vi "InvMP_Host_flatpotential.vi"() -> ()   [LabVIEW 2019]
uses:
  <vilib>/rvi/interface/nirviMethod/nirviMethod.xnode
  <vilib>/rvi/errors/niLvFpgaMergeErrorWithErrorCode.vi
  <vilib>/rvi/interface/nirviReadWriteControl/nirviReadWriteControl.xnode
  <vilib>/rvi/interface/Simulation/niFpgaSimulationCallBeginRW.vi
  <vilib>/rvi/errors/niLvFpgaAdjustHostInterfaceError.vi
  <vilib>/Utility/file.llb/Write Delimited Spreadsheet (DBL).vi
  <vilib>/Analysis/NI_AALBase.lvlib
  <vilib>/Analysis/baseanly.llb/Mean (DBL).vi
  <vilib>/FPGAPlugInAG/Dynamic/niLvFpga_Reset_Dynamic.vi
  <vilib>/FPGAPlugInAG/Dynamic/niLvFpga_Run_Dynamic.vi
  <vilib>/rvi/interface/nirviCloseFPGA/nirviCloseFPGA.xnode
  <vilib>/rvi/interface/nirviOpenFPGA/nirviOpenFPGA.xnode
  <vilib>/FPGAPlugInAG/Dynamic/niLvFpga_ConfigureFifo_Dynamic.vi
  <vilib>/FPGAPlugInAG/Dynamic/niLvFpga_StartFifo_Dynamic.vi
  <vilib>/FPGAPlugInAG/Dynamic/niLvFpga_ReadFifo_Dynamic.vi
  <vilib>/FPGAPlugInAG/Dynamic/niLvFpga_StopFifo_Dynamic.vi
  <vilib>/FPGAPlugInAG/Dynamic/niLvFpga_Close_Dynamic.vi
panel:
  in  "Menu Ring":u16(ring) items=["No FB", "HW", "FB"]
  out "Fx out":sgl=5.0307837
  in  "wait time":sgl=50.0
  in  "Fiting Control":enum32{"Fitting Control", "Fitting Errors"}(tab)
  out "signal\n offset_X":sgl=5.0
  in  "Fit?":bool
  out "best fit parameters":sgl[](array[numeric])=[0.33487067, 59.390804, 36.828644, -192.99852, -9974.326, 113441.81]
  out "residue":dbl
  in  "initial\nparameters":dbl[](array[numeric])=[0.0, 65.0, 0.0, -747.0, 30000.0, 300000.0, 0.0]
  in  "Offset":sgl=5.0
  out "Fitting in \nprogress":bool
  in  "Cal px/V":dbl=93.535 format="%#_13g"
  out "Pos array":sgl[](array[numeric])
  out "Volt":sgl[](array[numeric])
  out "error out":errorcluster
  out "smoothing error":i32
  in  "Calibration":T1={"K0"=0.0, "K1"=1.0, "K2"=0.0, "K3"=0.0, "K4"=0.0, "K5"=0.0}
  in  "Use Cal?":bool=TRUE
  in  "V_offset":sgl
  in  "Bias":sgl=0.0001
  in  "Xmin":sgl=-1.0
  in  "Fmax":sgl=100.0
  in  "Xmax":sgl=3.0
  out "num of protocols":sgl=1592.0
  in  "Calibration ON/OFF":bool=TRUE
  in  "Xoffset":sgl=0.00147
  in  "Yoffset":sgl=-0.00294
  in  "sum_offset":sgl=-0.0068
  in  "DW":cluster{"xm":sgl, "Eb":sgl, "Tau":sgl, "dE":sgl}={"xm"=0.5, "Eb"=0.005, "Tau"=80.0, "dE"=0.0} {"dE" format="%#_3g"}
  in  "DL_Y":dbl=2.5 format="%#_13g"
  in  "TL_Y":dbl=2.5 format="%#_13g"
  in  "STOP":bool
  in  "FB time":u32=10
  in  "Triangle wave":T2={"signal offset_X"=5.0, "Scale X"=0.0, "signal offset_Y"=5.0, "Scale Y"=0.0, "Phase Shift"=40}
  in  "Elements":u32=100000
  in  "Data length":dbl=20.0
  out "Done saving":bool
  out "?":dbl=-187.0
  in  "Save Data":bool
  in  "mobX(px/V)":sgl=1.0
  in  "1/Xcali":sgl=1.0
  in  "DX":sgl=51.12
  out "Feedback Loop time":sgl=10.0 format="%.2f"
  out "Underflow":bool
  out "X":waveform(dbl)(graph)={"t0"=timestamp(0 s since 1904-01-01), "dt"=9.999999747378752e-06, "Y"=array[100000 elements]}
  out "Y":waveform(dbl)(graph)={"t0"=timestamp(0 s since 1904-01-01), "dt"=9.999999747378752e-06, "Y"=array[100000 elements]}
  out "Sum":waveform(dbl)(graph)={"t0"=timestamp(0 s since 1904-01-01), "dt"=9.999999747378752e-06, "Y"=array[100000 elements]}
  in  "Reaverage PS":bool
  out "meanX":dbl=0.16896048917708206 format="%0.5f"
  in  "Xmean":sgl
  out "PSX":dynamicdata(graph)=[{"t0"=timestamp(0 s since 1904-01-01), "dt"=1.0000000252621255, "Y"=array[50000 elements], "attributes"=variant("NI_ChannelName"=variant(string "PSD"))}]
  out "PSY":dynamicdata(graph)=[{"t0"=timestamp(0 s since 1904-01-01), "dt"=1.0000000252621255, "Y"=array[50000 elements], "attributes"=variant("NI_ChannelName"=variant(string "PSD"))}]
  out "PSsum":dynamicdata(graph)=[{"t0"=timestamp(0 s since 1904-01-01), "dt"=1.0000000252621255, "Y"=array[50000 elements], "attributes"=variant("NI_ChannelName"=variant(string "PSD"))}]
  out "Saveloop":u32
  in  "Feedback parameters":T3={"SP_QPDX"=0.0, "alpha"=-0.1, "ktrap"=45.7534, "alphacounterX"=0.0218689}
  in  "TW freq":dbl=1.0
  in  "Normalize signal":bool=TRUE
  out "meanY":dbl=0.4494399424203283 format="%0.5f"
  out "meanZ":dbl=0.6937766502952576 format="%0.4f"
  out "?":errorcluster
  in  "file path (dialog if empty)":path=path "C:/Users/Diffusivity/Desktop/Inverse_Mpemba_starting June16/26-08-2020/t.txt"
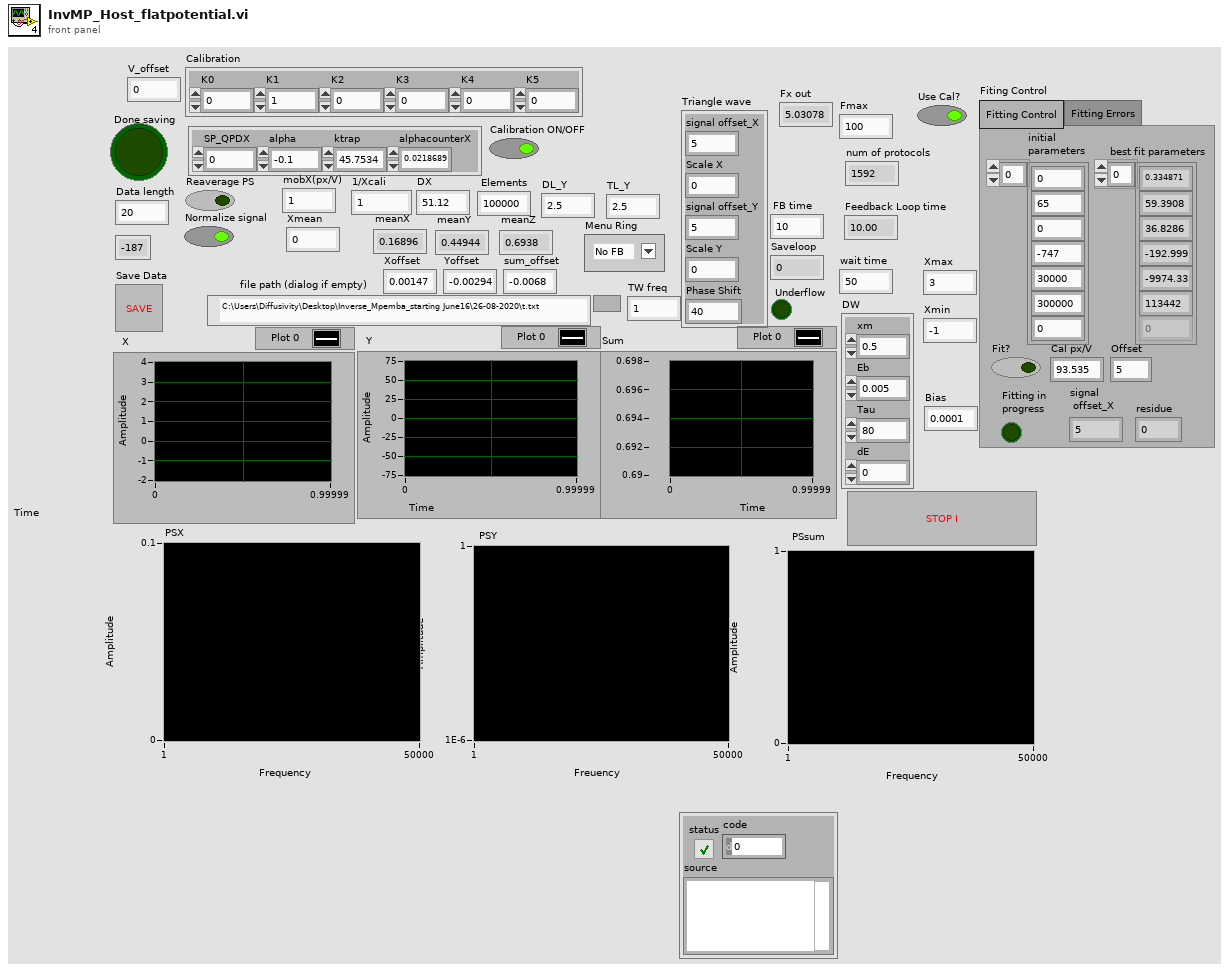
[diagram p1: front panel]
types:
  T1 = cluster{"K0":sgl, "K1":sgl, "K2":sgl, "K3":sgl, "K4":sgl, "K5":sgl}
  T2 = cluster{"signal offset_X":sgl, "Scale X":sgl, "signal offset_Y":sgl, "Scale Y":sgl, "Phase Shift":u32}
  T3 = cluster{"SP_QPDX":sgl, "alpha":sgl, "ktrap":sgl, "alphacounterX":sgl}
  T4 = cluster{"signal offset_X":sgl, "Scale X":sgl, "signal offset_Y":sgl, "Scale Y":sgl, u32}
  T5 = cluster{"[0]":sgl, "[1]":sgl, "[2]":sgl, "[3]":sgl, "[4]":sgl, "[5]":sgl}
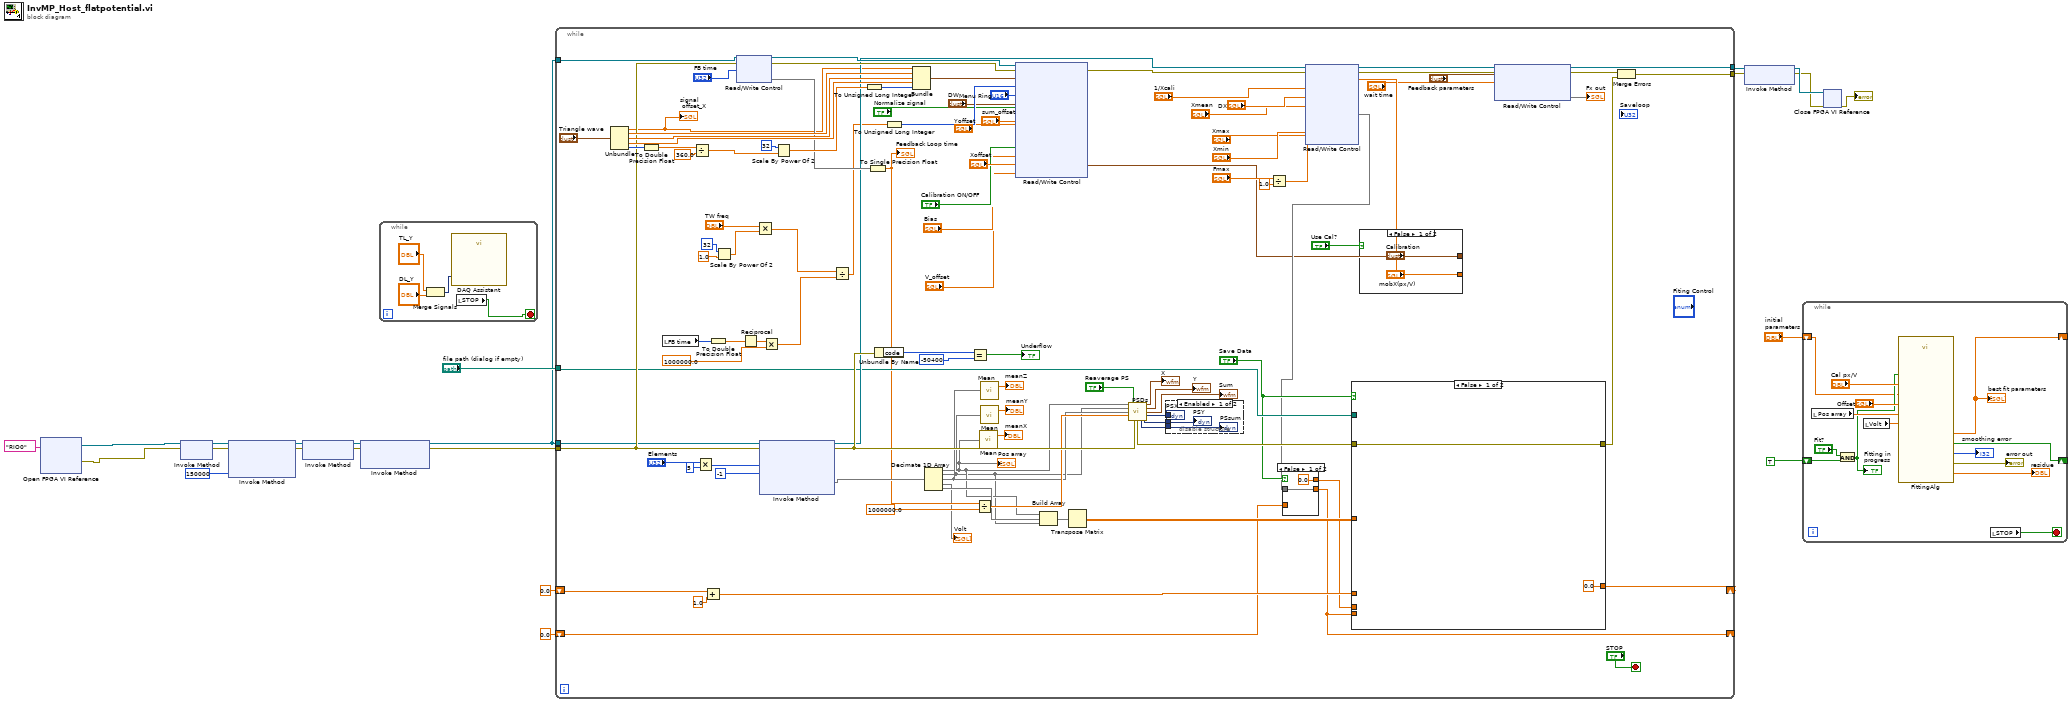
[diagram p0: block diagram]
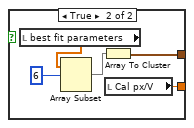
[diagram p2: hidden frame]
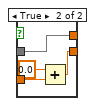
[diagram p3: hidden frame]
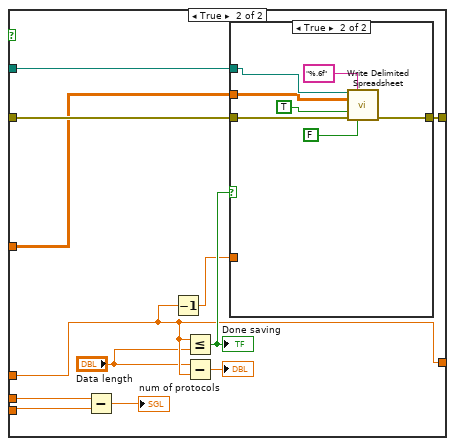
[diagram p5: hidden frame]
diagram:
  n1 = xnode "Open FPGA VI Reference"("resource name"=tag "RIO0") -> ("FPGA VI Reference Out"=w3:refnum<k20>, "error out"=w2:errorcluster)  [unwired: 1 in]
  n2 = xnode "Invoke Method"("FPGA VI Reference In"=w3, "error in"=w2) -> ("FPGA VI Reference Out"=w12:refnum<k20>, "error out"=w11:errorcluster)
  n3 = xnode "Invoke Method"("FPGA VI Reference In"=w12, "error in"=w11, "Requested Depth"=u32 150000) -> ("FPGA VI Reference Out"=w17:refnum<k20>, "error out"=w16:errorcluster)  [unwired: 1 out]
  n4 = xnode "Invoke Method"("FPGA VI Reference In"=w17, "error in"=w16) -> ("FPGA VI Reference Out"=w19:refnum<k20>, "error out"=w18:errorcluster)
  n5 = xnode "Invoke Method"("FPGA VI Reference In"=w19, "error in"=w18) -> ("FPGA VI Reference Out"=w15:refnum<k20>, "error out"=w14:errorcluster)  [unwired: 1 in]
  n6 = while {
    stop <- w23 stop-if-true
    n7 = Merge Signals("TL_Y", "DL_Y") -> (w26:dynamicdata)
    n8 = call "DAQ Assistant"("data"=w26) -> ()  [unwired: 17 in, 2 out]
    n9 = local read "STOP"() -> (w23:bool)
  }
  n10 = while {
    tunnel: w15 -> [w106]
    tunnel: w14 -> [w107]
    tunnel: "file path (dialog if empty)" -> [w76]
    tunnel: [w99] -> w21
    tunnel: [w112] -> w20
    tunnel: w15 -> [w94]
    shift-right: [w103] -> _
    shift-left: 0.0 -> [w102]
    shift-right: [w45] -> _
    shift-left: sgl 0.0 ("num of cycles") -> [w47]
    stop <- "STOP" stop-if-true
    n11 = Unbundle("Triangle wave") -> ("signal offset_X"=w33:sgl, "Scale X"=w116:sgl, "signal offset_Y"=w115:sgl, "Scale Y"=w114:sgl, "Phase Shift"=w117:u32)
    "signal\n offset_X" <- w33
    n12 = To Double Precision Float(number=w117) -> (double precision float=w123:dbl)
    n13 = local read "FB time"() -> (w66:u32)
    n14 = Divide(x=w123, y=360.0) -> (x/y=w121:dbl)
    n15 = Multiply(x="Elements", y=u32 5) -> (x*y=w108:u32)
    n16 = Add(x=w102, y=1.0) -> (x+y=w104:dbl)
    n17 = To Double Precision Float(number=w66) -> (double precision float=w67:dbl)
    n18 = Scale By Power Of 2(n=i16 32, x=1.0) -> (x*2^n=w71:dbl)
    n19 = xnode "Read/Write Control"("FPGA VI Reference In"=w106, "error in"=w107, "FB Time"="FB time") -> ("FPGA VI Reference Out"=w128:refnum<k20>, "error out"=w95:errorcluster, "FB Time"=w93)
    n20 = Reciprocal(x=w67) -> (1/x=w68:dbl)
    n21 = Multiply(x="TW freq", y=w71) -> (x*y=w64:dbl)
    n22 = xnode "Invoke Method"("FPGA VI Reference In"=w94, "error in"=w107, "Number of Elements"=w108, "Timeout (ms)"=-1) -> ("FPGA VI Reference Out"=w78:refnum<k20>, "error out"=w91:errorcluster, "Data"=w87:void[])  [unwired: 1 out]
    n23 = Multiply(x=w68, y=1000000.0) -> (x*y=w63:dbl)
    n24 = Scale By Power Of 2(n=i16 32, x=w121) -> (x*2^n=w119:dbl)
    n25 = Divide(x=w64, y=w63) -> (x/y=w62:dbl)
    n26 = To Unsigned Long Integer(number=w119) -> (unsigned 32bit integer=w113:u32)
    n27 = To Single Precision Float(number=w93) -> (single precision float=w73:sgl)
    "Feedback Loop time" <- w73
    n28 = Unbundle By Name(w91) -> ("code"=w111:i32)
    n29 = To Unsigned Long Integer(number=w62) -> (unsigned 32bit integer=w61:u32)
    n30 = Bundle("signal offset_X"=w33, "Scale X"=w116, "signal offset_Y"=w115, "Scale Y"=w114, w113) -> (w74:T4)  [unwired: 1 in]
    n31 = Decimate 1D Array(w87) -> (w35:void[], w27:void[], w54:void[], →"Volt":void[], w55:void[])
    "Pos array" <- w35
    n32 = Equal?(x=w111, y=-50400) -> (x = y?=→"Underflow":bool)
    n33 = Divide(x=w73, y=sgl 1000000.0) -> (x/y=w56:sgl)
    n34 = call-poly <vilib>:"Mean.vi"("X"=w35) -> ("mean"=→"meanX":dbl)  [unwired: 1 out]
    n35 = call-poly <vilib>:"Mean.vi"("X"=w54) -> ("mean"=→"meanZ":dbl)  [unwired: 1 out]
    n36 = call-poly <vilib>:"Mean.vi"("X"=w27) -> ("mean"=→"meanY":dbl)  [unwired: 1 out]
    n37 = Build Array(w35, w55, w27) -> (w97:void[])
    n38 = Transpose Matrix(1:w97) -> (0:w126:dbl[][])
    n39 = call "PSDs.vi"("X"=w35, "averaging done"="Reaverage PS", "Y"=w27, "sum"=w54, "dt"=w56, "error in (no error)"=w91) -> ("X"=→"X":waveform(dbl), "Y"=→"Y":waveform(dbl), "Sum"=→"Sum":waveform(dbl), "PSDX"=w83:dynamicdata, "error out"=w90:errorcluster, "PSDsum"=w81:dynamicdata, "PSDY"=w82:dynamicdata)  [unwired: 3 in]
    n40 = disable-structure shown="Enabled" {
      disable-tunnel: w83 -> [w146 _]
      disable-tunnel: w82 -> [w145 _]
      disable-tunnel: w81 -> [w144 _]
      frame Enabled {
        "PSX" <- w146
        "PSY" <- w145
        "PSsum" <- w144
      }
      frame Disabled {
      }
    }
    n41 = Divide(x="Fmax", y=sgl 1.0) -> (x/y=w42:sgl)
    n42 = case shown="False" "Use Cal?" {
      tunnel: ["Calibration" w137] -> w37
      tunnel: ["mobX(px/V)" w134] -> w36
      frame False {
      }
      frame True {
        n43 = local read "best fit parameters"() -> (w133:sgl[])
        n44 = Array Subset(array=w133, length=6) -> (w135:sgl[])  [unwired: 1 in]
        n45 = Array To Cluster(array=w135) -> (cluster=w137:T5)
        n46 = local read "Cal px/V"() -> (w134:dbl)
      }
    }
    n47 = xnode "Read/Write Control"("FPGA VI Reference In"=w128, "error in"=w95, "Triangle wave"=w74, "Frequency"=w61, "Enum"="Menu Ring", "DW"="DW", "Normalize signal"="Normalize signal", "sum_offset"="sum_offset", "Yoffset"="Yoffset", "Xoffset"="Xoffset", "Calibration ON/OFF"="Calibration ON/OFF", "Bias"="Bias", "Calibration"=w37, "V_offset"="V_offset") -> ("error out"=w77:errorcluster)  [unwired: 1 out]
    n48 = xnode "Read/Write Control"("FPGA VI Reference In"=w78, "error in"=w77, "MobX(px/V)"=w36, "1/Xcali"="1/Xcali", "DX"="DX", "Xmean"="Xmean", "Fmax"=w42, "Xmin"="Xmin", "Xmax"="Xmax") -> ("FPGA VI Reference Out"=w101:refnum<k20>, "error out"=w100:errorcluster, "num of cycles"=w44)
    n49 = case shown="False" "Save Data" {
      tunnel: w44 -> [w139 w140]
      tunnel: [w139 w141] -> w45
      tunnel: w47 -> [_ w142]
      tunnel: [sgl 0.0 ("num of cycles") w140] -> w46
      frame False {
      }
      frame True {
        n50 = Add(x=sgl 0.0 ("num of cycles"), y=w142) -> (x+y=w141:sgl)
      }
    }
    n51 = case shown="False" "Save Data" {
      tunnel: w126 -> [_ w155]
      tunnel: w76 -> [_ w160]
      tunnel: w90 -> [w148 w159]
      tunnel: [w148 w158] -> w125
      tunnel: w104 -> [_ w154]
      tunnel: [0.0 w154] -> w103
      tunnel: w46 -> [_ w151]
      tunnel: w45 -> [_ w150]
      frame False {
      }
      frame True {
        n52 = Subtract(x=w151, y=w150) -> (x-y=→"num of protocols":sgl)
        n53 = Decrement(x=w154) -> (x-1=w153:dbl)
        n54 = Less Or Equal?(x=w154, y="Data length") -> (x <= y?=w157:bool)
        "Done saving" <- w157
        n55 = Subtract(x="Data length", y=w154) -> (x-y=→"?":dbl)
        n56 = case shown="True" w157 {
          tunnel: w155 -> [_ w162]
          tunnel: w160 -> [_ w163]
          tunnel: w159 -> [w161 w166]
          tunnel: [w161 w165] -> w158
          tunnel: w153 -> [_ _]
          frame False {
          }
          frame True {
            n57 = call-poly <vilib>:"Write Delimited Spreadsheet.vi"("file path (dialog if empty)"=w163, "format (%.3f)"="%.6f", "2D data"=w162, "append to file? (new file:F)"=TRUE, "error in (no error)"=w166, "transpose? (no:F)"=FALSE) -> ("error out"=w165:errorcluster)  [unwired: 8 in, 1 out]
          }
        }
      }
    }
    n58 = xnode "Read/Write Control"("FPGA VI Reference In"=w101, "error in"=w100, "Feedback parameters"="Feedback parameters", "wait time"="wait time") -> ("FPGA VI Reference Out"=w99:refnum<k20>, "error out"=w98:errorcluster, "Fx out"=→"Fx out")
    n59 = Merge Errors(w98, w125) -> (w112:errorcluster)
  }
  n60 = xnode "Invoke Method"("FPGA VI Reference In"=w21, "error in"=w20) -> ("FPGA VI Reference Out"=w10:refnum<k20>, "error out"=w9:errorcluster)
  n61 = while {
    shift-right: [w174] -> _
    shift-left: TRUE -> [w175]
    shift-right: [w170] -> _
    shift-left: "initial\nparameters" -> [w169]
    stop <- w181 stop-if-true
    n62 = local read "Pos array"() -> (w180:sgl[])
    n63 = And(x="Fit?", y=w175) -> (x .and. y?=w173:bool)
    "Fitting in \nprogress" <- w173
    n64 = local read "Volt"() -> (w179:sgl[])
    n65 = call "FittingAlg.vi"("Pos"=w180, "Cal px/V"="Cal px/V", "initial parameters"=w169, "Volt"=w179, "Boolean in"=w173, "Offset"="Offset") -> ("error"=→"smoothing error":i32, "best fit parameters"=w170:dbl[], "Boolean out"=w174:bool, "residue"=→"residue":dbl, "error out"=→"error out":errorcluster)  [unwired: 5 in]
    "best fit parameters" <- w170
    n66 = local read "STOP"() -> (w181:bool)
  }
  n67 = xnode "Close FPGA VI Reference"("FPGA VI Reference In"=w10, "error in"=w9) -> ("error out"=→"?":errorcluster)
